vi "to string array.vi"(8 "error in (no error)":errorcluster, 11 "Increment configuration in":refnum<class "Increment configuration.lvclass">) -> (0 "error out":errorcluster, 1 "Array":string[][](array[string]), 2 "version":string, 3 "Increment configuration out":refnum<class "Increment configuration.lvclass">)   [LabVIEW 2015, in "Increment configuration.lvclass"]
uses:
  Increment configuration.lvclass
  Increment configuration.lvclass/Increment configuration.ctl
  Read Lines.vi
  <vilib>/NI/Tag Bus Module Framework/channel/TBM channel.lvclass
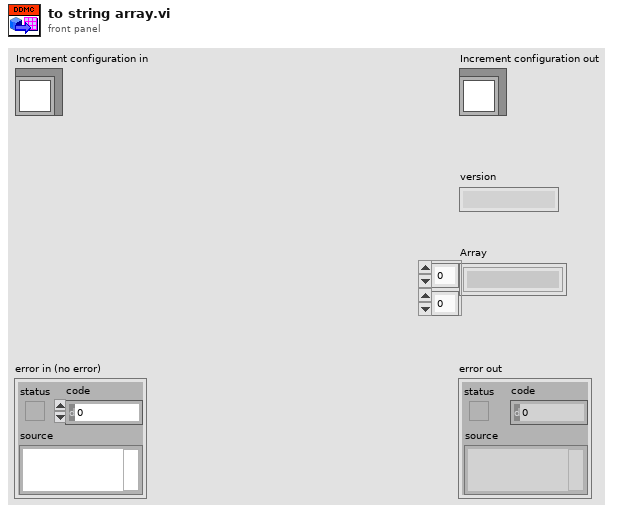
[diagram p1: front panel]
types:
  T1 = typedef "Increment configuration.lvclass/Line.ctl" = cluster{"Name":string, "channel in":refnum<class "TBM channel.lvclass">, "channel out":refnum<class "TBM channel.lvclass">}
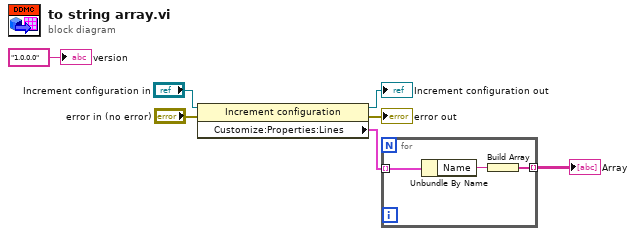
[diagram p0: block diagram]
diagram:
  n1 = property class="Increment configuration"(reference="Increment configuration in", error in="error in (no error)") -> (reference out=→"Increment configuration out":refnum<class "Increment configuration.lvclass">, error out=→"error out":errorcluster, "Customize:Properties:Lines"=w4:T1[])
  n2 = for {
    tunnel: w4 -> [w10] mode=indexing
    tunnel: [w9] -> w1 mode=indexing
    n3 = Unbundle By Name(w10) -> ("Name"=w8:string)
    n4 = Build Array(w8) -> (w9:string[])
  }
  "Array" <- w1
  "version" <- "1.0.0.0" ("version")
